vi "array page down.vi"(8 "error in (no error)":errorcluster, 11 "Array in":refnum<vi>) -> (0 "error out":errorcluster, 3 "Array out":refnum<vi>)   [LabVIEW 2014, in "Tagbus PID Module editor node.lvclass"]
uses:
  Tagbus PID Module editor node.lvclass
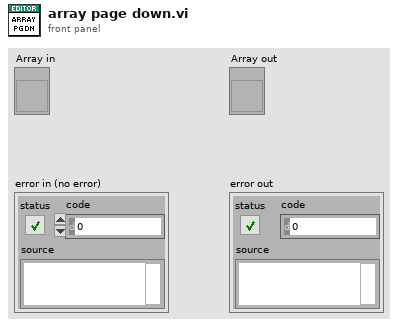
[diagram p1: front panel]
types:
  T1 = cluster{"Loop ID":string, "Tags":cluster{"Setpoint":string, "Process Variable":string, "Output":string}, "Gains":cluster{"P":dbl, "I":dbl, "D":dbl}, "Range":cluster{"High":dbl, "Low":dbl}}[]
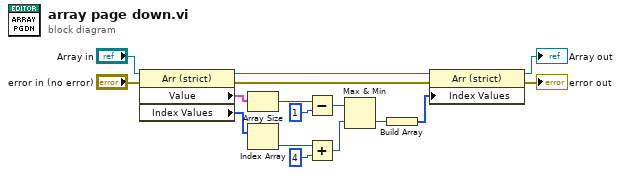
[diagram p0: block diagram]
diagram:
  n1 = property class="Arr (strict)"(reference="Array in", error in="error in (no error)") -> (reference out=w4:refnum<vi>, error out=w13:errorcluster, "Value"=w12:T1, "Index Values"=w6:u32[])
  n2 = Array Size(array=w12) -> (size(s)=w3:i32)
  n3 = Index Array(array=w6) -> (element=w7:u32)  [unwired: 1 in]
  n4 = Subtract(x=w3, y=u32 1) -> (x-y=w1:u32)
  n5 = Add(x=w7, y=u32 4) -> (x+y=w9:u32)
  n6 = Max & Min(x=w1, y=w9) -> (min(x,y)=w11:u32)  [unwired: 1 out]
  n7 = Build Array(w11) -> (w10:u32[])
  n8 = property class="Arr (strict)"(reference=w4, error in=w13, "Index Values"=w10) -> (reference out=→"Array out":refnum<vi>, error out=→"error out":errorcluster)
